vi "Parse Data JSON.vi"(8 "error in (no error)":errorcluster, 10 "JSON String":string, 11 "Hello in":refnum<class "Hello.lvclass">) -> (0 "error out":errorcluster, 1 "Typed?":bool, 2 "Typed Message":refnum<class "Response.lvclass">, 3 "Hello out":refnum<class "Hello.lvclass">)   [LabVIEW 2022 SP3, in "obs-websocket-lv.lvlib" / "Hello.lvclass"]
uses:
  Hello.lvclass
  Response/Response.lvclass
  Authentication.ctl
  Hello.lvclass/Hello.ctl
  <vilib>/IlluminatedG/lv-web-crypto/lv-json/JSON/JSON.lvlib
  obs-websocket-lv.lvlib
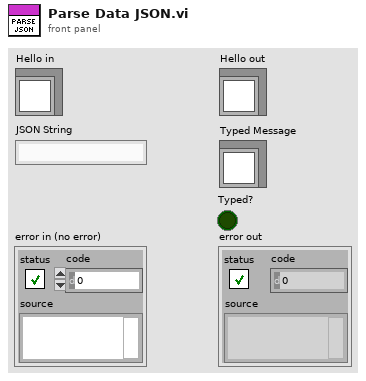
[diagram p1: front panel]
types:
  T1 = typedef "JSON.lvlib/JSON Item Type.ctl" = enum16{"unknown", "null", "Array", "Object", "String", "Number", "Boolean"}
  T2 = typedef "obs-websocket-lv.lvlib/Authentication.ctl" = cluster{"Has Authentication":bool, "Salt":string, "Challenge":string}
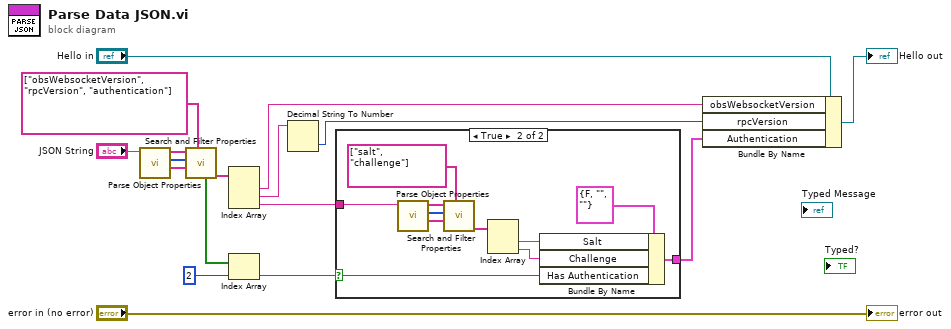
[diagram p0: block diagram]
diagram:
  n1 = call <vilib>:"Parse Object Properties.vi"("JSON String"="JSON String") -> ("Values"=w13:string[], "Item Types"=w14:T1[], "Keys"=w15:string[])  [unwired: 7 in, 1 out]
  n2 = call <vilib>:"Search and Filter Properties.vi"("Search Keys"=string[] ["obsWebsocketVersion", "rpcVersion", "authentication"], "Values In"=w13, "Types In"=w14, "Keys In"=w15) -> ("Filtered Values"=w11:string[], "Item Found"=w9:bool[])  [unwired: 2 in, 4 out]
  n3 = Index Array(array=w11) -> (element #1=w8:string, element #2=w7:string, element #3=w4:string)  [unwired: 3 in]
  n4 = Index Array(array=w9, index=2) -> (element=w5:bool)
  n5 = Decimal String To Number(string=w7) -> (number=w6:i32)  [unwired: 2 in, 1 out]
  n6 = case shown="True" w5 {
    selector: w5 -> [_ w19]
    tunnel: w4 -> [_ w28]
    tunnel: [_ w18] -> w1
    frame False {
    }
    frame True {
      n7 = call <vilib>:"Parse Object Properties.vi"("JSON String"=w28) -> ("Values"=w25:string[], "Item Types"=w26:T1[], "Keys"=w27:string[])  [unwired: 7 in, 1 out]
      n8 = call <vilib>:"Search and Filter Properties.vi"("Search Keys"=string[] ["salt", "challenge"], "Values In"=w25, "Types In"=w26, "Keys In"=w27) -> ("Filtered Values"=w23:string[])  [unwired: 2 in, 5 out]
      n9 = Index Array(array=w23) -> (element #1=w21:string, element #2=w20:string)  [unwired: 2 in]
      n10 = Bundle By Name(cluster=T2 {"Has Authentication"=FALSE, "Salt"="", "Challenge"=""} ("Authentication"), "Salt"=w21, "Challenge"=w20, "Has Authentication"=w19) -> (w18:T2)
    }
  }
  n11 = Bundle By Name(cluster="Hello in", "obsWebsocketVersion"=w8, "rpcVersion"=w6, "Authentication"=w1) -> (→"Hello out":refnum<class "Hello.lvclass">)
  "error out" <- "error in (no error)"
